vi "RunVI.vi"(0 "VI Ref In":refnum<vi>, 11 "Error In":errorcluster) -> (4 "VI Ref Out":refnum<vi>, 15 "Error Out":errorcluster)   [LabVIEW 2019, in "JsonToCluster.lvlib"]
doc: "This VI runs the given VI reference"
uses:
  JsonToCluster.lvlib
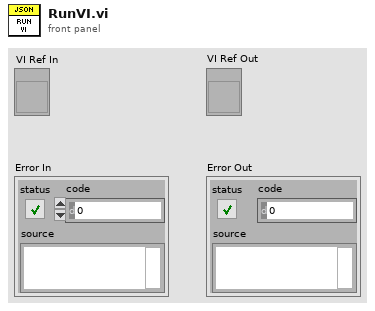
[diagram p1: front panel]
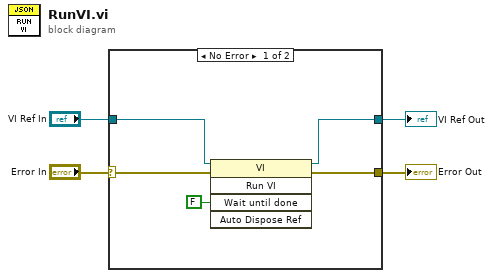
[diagram p0: block diagram]
diagram:
  n1 = case shown="No Error" "Error In" {
    selector: "Error In" -> [w7 w11]
    tunnel: [w9 w11] -> w2
    tunnel: "VI Ref In" -> [w6 w10]
    tunnel: [w5 w10] -> w1
    frame No Error {
      n2 = invoke class="VI" method="Run VI"(reference=w6, error in=w7, "Wait until done"=FALSE ("Wait Until Done")) -> (reference out=w5:refnum<vi>, error out=w9:errorcluster)  [unwired: 2 in, 3 out]
    }
    frame Error {
    }
  }
  "Error Out" <- w2
  "VI Ref Out" <- w1
